vi "Config Socket.vi"(8 "error in (no error)":errorcluster, 10 "Socket Config":T1={"Socket"=refnum, "socket type"=enum."ZMQ_PUB", "endpoint"="tcp://*:5555", "filter"=""}, 11 "ZMQ in":refnum<class "RemoteControl.ZMQ.lvclass">) -> (0 "error out":errorcluster, 3 "ZMQ out":refnum<class "RemoteControl.ZMQ.lvclass">)   [LabVIEW 2019, in "RemoteControl.ZMQ.lvclass"]
uses:
  RemoteControl.ZMQ.lvclass
  <vilib>/addons/zeromq/socket_type.ctl
  <vilib>/addons/zeromq/zeromq.lvlib
  Typedefs/ZMQ Config.ctl
  <vilib>/addons/zeromq/zmq_socket.lvclass
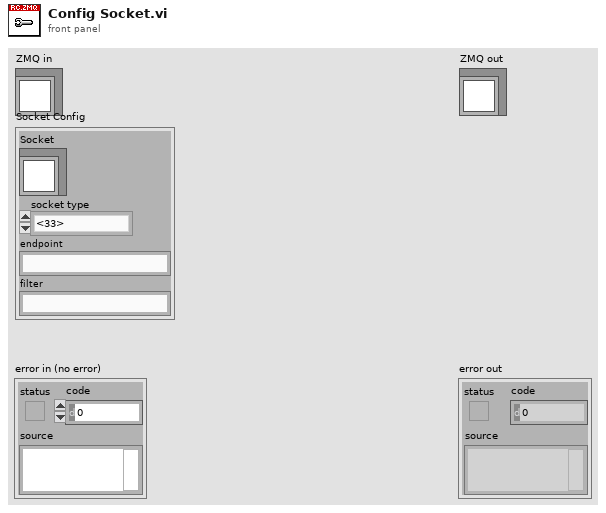
[diagram p1: front panel]
types:
  T1 = typedef "RemoteControl.ZMQ.lvclass/ZMQ Config.ctl" = cluster{"Socket":refnum<class "zmq_socket.lvclass">, "socket type":T2, "endpoint":string, "filter":string}
  T2 = typedef "zeromq.lvlib/socket_type.ctl" = enum8{"ZMQ_PAIR", "ZMQ_PUB", "ZMQ_SUB", "ZMQ_REQ", "ZMQ_REP", "ZMQ_DEALER", "ZMQ_ROUTER", "ZMQ_PULL", "ZMQ_PUSH", "ZMQ_XPUB", "ZMQ_XSUB"}
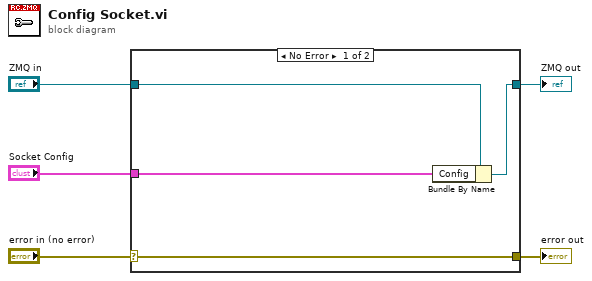
[diagram p0: block diagram]
diagram:
  n1 = case shown="No Error" "error in (no error)" {
    selector: "error in (no error)" -> [w9 w10]
    tunnel: [w9 w10] -> w4
    tunnel: [w7 w11] -> w2
    tunnel: "ZMQ in" -> [w8 w11]
    tunnel: "Socket Config" -> [w6 _]
    frame No Error {
      n2 = Bundle By Name(cluster=w8, "Config"=w6) -> (w7:refnum<class "RemoteControl.ZMQ.lvclass">)
    }
    frame Error {
    }
  }
  "error out" <- w4
  "ZMQ out" <- w2
